vi "permutcolon.vi"(11 "Cell Voltages en entrée":dbl[][](array[numeric])) -> (3 "tableau en sortie":dbl[][](array[numeric]))   [LabVIEW 2020]
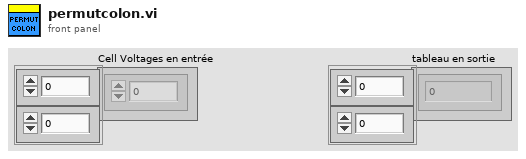
[diagram p1: front panel]
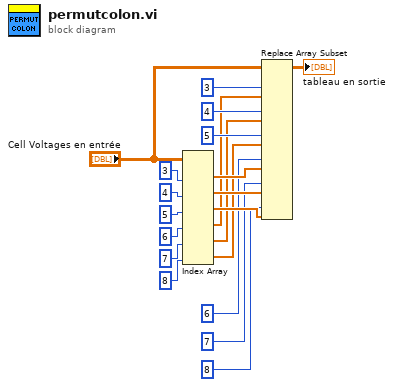
[diagram p0: block diagram]
diagram:
  n1 = Index Array(array="Cell Voltages en entrée", index (col) #1=3 ("indice désactivé (col)"), index (col) #2=4 ("indice (col)"), index (col) #3=5 ("indice (col)"), index (col) #4=6 ("indice (col)"), index (col) #5=7 ("indice (col)"), index (col) #6=8 ("indice (col)")) -> (element #1=w17:dbl[], element #2=w18:dbl[], element #3=w20:dbl[], element #4=w10:dbl[], element #5=w12:dbl[], element #6=w14:dbl[])  [unwired: 6 in]
  n2 = Replace Array Subset(array="Cell Voltages en entrée", new element #1=w10, index (col) #1=3 ("indice désactivé (col)"), new element #2=w12, index (col) #2=4 ("indice (col)"), new element #3=w14, index (col) #3=5 ("indice (col)"), new element #4=w17, index (col) #4=6 ("indice (col)"), new element #5=w18, index (col) #5=7 ("indice (col)"), new element #6=w20, index (col) #6=8 ("indice (col)")) -> (→"tableau en sortie":dbl[][])  [unwired: 6 in]
